vi "myRIO_BRig_RT_dataCurrent_CueLed_pulse_duration.vi"() -> (2 "output_CueLed_pulse_duration":i32)   [LabVIEW 2014]
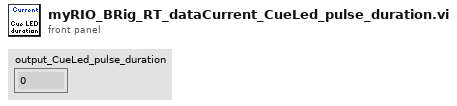
[diagram p1: front panel]
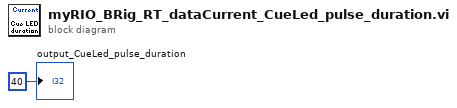
[diagram p0: block diagram]
diagram:
  "output_CueLed_pulse_duration" <- 40 ("output_iBlock")
